vi "Check if configuration files exist.vi"(8 "error in (no error)":errorcluster, 11 "DAQCascade512Base in":refnum<class "DAQCascade512.lvclass">) -> (0 "error out":errorcluster, 2 "configuration file exists?":bool, 3 "DAQCascade512Base out":refnum<class "DAQCascade512.lvclass">)   [LabVIEW 2012, in "DAQCascade512.lvclass"]
doc: "Checks whether all required configuration files for the component tree exists."
uses:
  DAQCascade512.lvclass
  <vilib>/Distrio/Murmex/Murmex/Murmex.lvclass
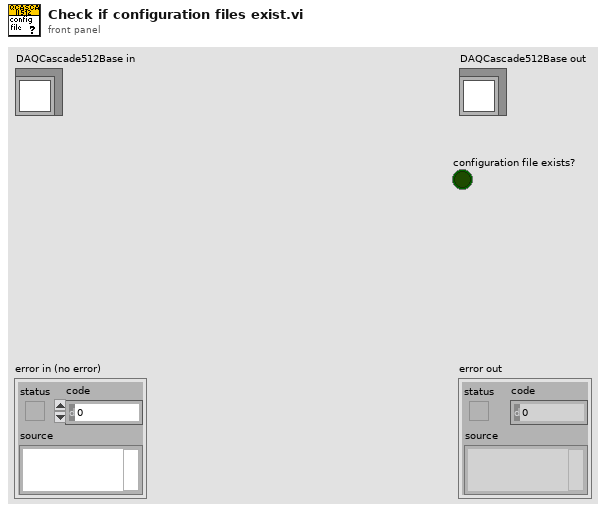
[diagram p1: front panel]
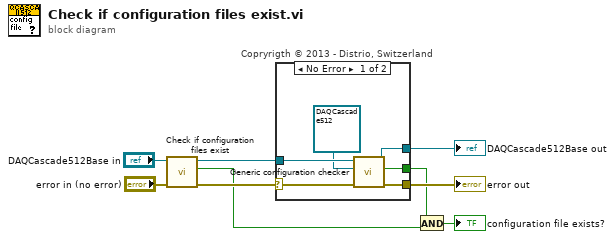
[diagram p0: block diagram]
diagram:
  n1 = call-parent "Check if configuration files exist.vi"("error in (no error)"="error in (no error)", "MurmexBase in"="DAQCascade512Base in") -> ("error out"=w6:errorcluster, "configuration file exists?"=w1:bool, "MurmexBase out"=w3:refnum<class "DAQCascade512.lvclass">)  [unwired: 7 in]
  "error out" <- w6
  n2 = case "Copryrigth © 2013 - Distrio, Switzerland" shown="No Error" w6 {
    selector: w6 -> [w14 w16]
    tunnel: [w12 w16] -> _
    tunnel: [w10 w15] -> w2
    tunnel: w3 -> [w13 w15]
    tunnel: [w11 _] -> w5
    frame No Error {
      n3 = call <vilib>:"Generic configuration checker.vi"("error in (no error)"=w14, "inheritance level"=refnum<class "DAQCascade512.lvclass"> refnum ("DAQCascade512"), "Murmex in"=w13) -> ("error out"=w12:errorcluster, "configuration file exists?"=w11:bool, "Murmex out"=w10:refnum<class "DAQCascade512.lvclass">)  [unwired: 6 in]
    }
    frame Error {
    }
  }
  "DAQCascade512Base out" <- w2
  n4 = And(x=w5, y=w1) -> (x .and. y?=→"configuration file exists?":bool)
